vi "Plot_trap_heating_global_BM.vi"() -> ()   [LabVIEW 2021]
panel:
  out "Plot trap heating":bool
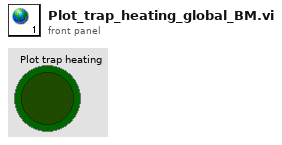
[diagram p1: front panel]
diagram:
